vi "Edit Target Settings_Edit.vi"(8 "error in (no error)":errorcluster, 10 "Settings":T1={"Name"="", "Target Type"="", "IPAddress"="localhost", "PrimaryControlLoopProcessor"=-2, "DataProcessingLoopProcessor"=-2, "DataProcessingLoopDecimation"=1, "DAQDigitalLinesDecimation"=1, "MaximumStreamedChannels"=512, "ExecutionMode"=0, "FilterDAQErrors"=FALSE, "FilterWatchdogErrors"=FALSE, "FPGAScanInterfaceMode"=0, "TargetRate"=0.0} {"FPGAScanInterfaceMode" items=["Use Current", "FPGA Mode", "Scan Mode"]; "ExecutionMode" items=["Parallel", "LowLatency"]}, 11 "Target Ref":refnum<k24>) -> (0 "error out":errorcluster, 3 "Target Ref Out":refnum<k24>)   [LabVIEW 2019, in "Simple SysDef API.lvlib"]
uses:
  <userlib>/SimpleSysDef/Simple SysDef API.lvlib
  <userlib>/SimpleSysDef/_SubVIs/Add Target_Settings.ctl
  <userlib>/SimpleSysDef/_SubVIs/Add Target_Types.ctl
  NationalInstruments.VeriStand.SystemDefinitionAPI
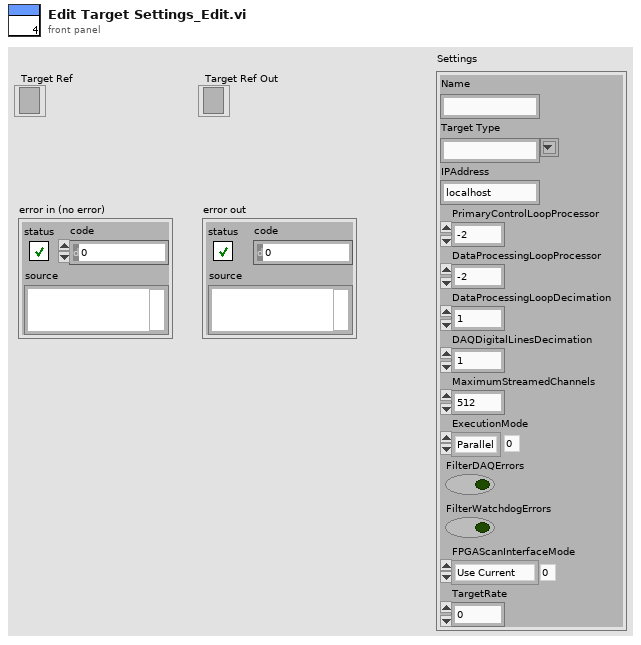
[diagram p1: front panel]
types:
  T1 = typedef "Simple SysDef API.lvlib/Add Target_Settings.ctl" = cluster{"Name":string, "Target Type":T2, "IPAddress":string, "PrimaryControlLoopProcessor":i32, "DataProcessingLoopProcessor":i32, "DataProcessingLoopDecimation":i32, "DAQDigitalLinesDecimation":u32, "MaximumStreamedChannels":i32, "ExecutionMode":i32, "FilterDAQErrors":bool, "FilterWatchdogErrors":bool, "FPGAScanInterfaceMode":u16, "TargetRate":dbl}
  T2 = typedef "Simple SysDef API.lvlib/Add Target_Types.ctl" = string
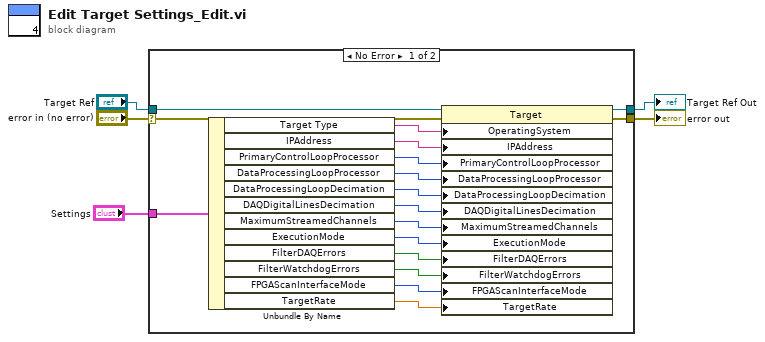
[diagram p0: block diagram]
diagram:
  n1 = case shown="No Error" "error in (no error)" {
    selector: "error in (no error)" -> [w8 w24]
    tunnel: "Settings" -> [w22 _]
    tunnel: [w21 w23] -> w4
    tunnel: "Target Ref" -> [w20 w23]
    tunnel: [w19 w24] -> w2
    frame No Error {
      n2 = Unbundle By Name(w22) -> ("Target Type"=w6:T2, "IPAddress"=w7:string, "PrimaryControlLoopProcessor"=w18:i32, "DataProcessingLoopProcessor"=w17:i32, "DataProcessingLoopDecimation"=w16:i32, "DAQDigitalLinesDecimation"=w15:u32, "MaximumStreamedChannels"=w14:i32, "ExecutionMode"=w13:i32, "FilterDAQErrors"=w12:bool, "FilterWatchdogErrors"=w11:bool, "FPGAScanInterfaceMode"=w10:u16, "TargetRate"=w9:dbl)
      n3 = property class="Target"(reference=w20, error in=w8, "OperatingSystem"=w6, "IPAddress"=w7, "PrimaryControlLoopProcessor"=w18, "DataProcessingLoopProcessor"=w17, "DataProcessingLoopDecimation"=w16, "DAQDigitalLinesDecimation"=w15, "MaximumStreamedChannels"=w14, "ExecutionMode"=w13, "FilterDAQErrors"=w12, "FilterWatchdogErrors"=w11, "FPGAScanInterfaceMode"=w10, "TargetRate"=w9) -> (reference out=w21:refnum<k24>, error out=w19:errorcluster)
    }
    frame Error {
    }
  }
  "Target Ref Out" <- w4
  "error out" <- w2
